vi "error.handler.vi"(8 "error in (no error)":errorcluster, 11 "comic_crawler in":refnum<class "comic_crawler.lvclass">) -> (0 "error out":errorcluster, 3 "comic_crawler out":refnum<class "comic_crawler.lvclass">, 4 "critical":bool)   [LabVIEW 2024, in "comic_crawler.lvclass"]
uses:
  comic_crawler.lvclass
  daemon.states--enum.ctl
  comic_crawler.lvclass/comic_crawler.ctl
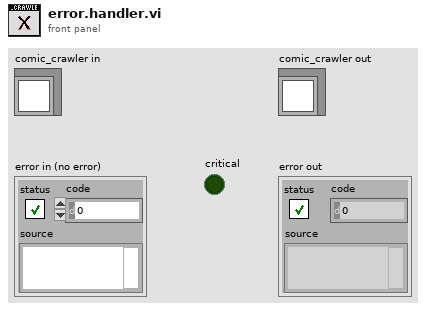
[diagram p1: front panel]
types:
  T1 = typedef "comic_crawler.lvclass/daemon.states--enum.ctl" = enum16{"start search", "idle", "set timer", "running", "stop search", "wait", "set delay", "shut down"}
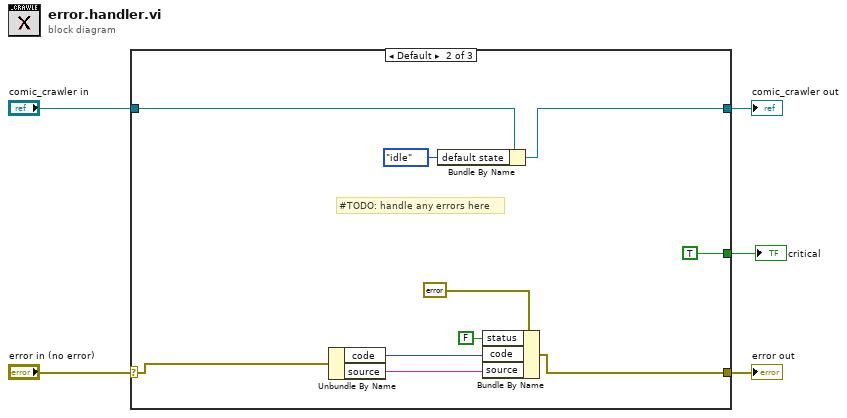
[diagram p0: block diagram]
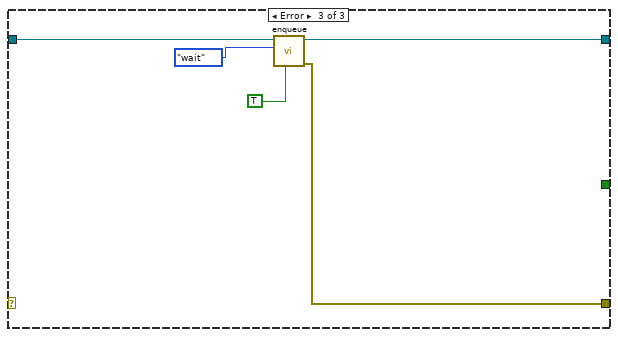
[diagram p3: hidden frame]
diagram:
  n1 = case shown="Default" "error in (no error)" {
    selector: "error in (no error)" -> [w6 w13 _]
    tunnel: [w6 w8 w18] -> w4
    tunnel: [w7 w14 w21] -> w2
    tunnel: "comic_crawler in" -> [w7 w16 w22]
    tunnel: [_ TRUE _] -> w1
    frame No Error {
    }
    frame Default {
      # "#TODO: handle any errors here"
      n2 = Unbundle By Name(w13) -> ("code"=w11:i32, "source"=w10:string)
      n3 = Bundle By Name(cluster=w16, "default state"=daemon.states--enum."idle") -> (w14:refnum<class "comic_crawler.lvclass">)
      n4 = Bundle By Name(cluster=errorcluster {"status"=FALSE, "code"=0, "source"=""} ("error IO"), "status"=FALSE, "code"=w11, "source"=w10) -> (w8:errorcluster)
    }
    frame Error {
      n5 = call "enqueue.vi"("priority (f)"=TRUE, "cmd"=daemon.states--enum."wait", "comic_crawler in"=w22) -> ("error out"=w18:errorcluster, "comic_crawler out"=w21:refnum<class "comic_crawler.lvclass">)  [unwired: 7 in]
    }
  }
  "error out" <- w4
  "comic_crawler out" <- w2
  "critical" <- w1
